vi "DELETE_req_PS.vi"(8 "error in":errorcluster, 10 "URL":string, 11 "Headers":string) -> (0 "error out":errorcluster, 3 "DELETE Request":string)   [LabVIEW 2016]
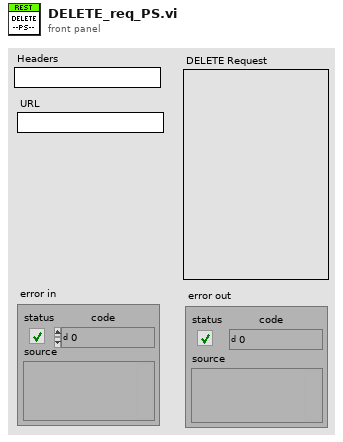
[diagram p1: front panel]
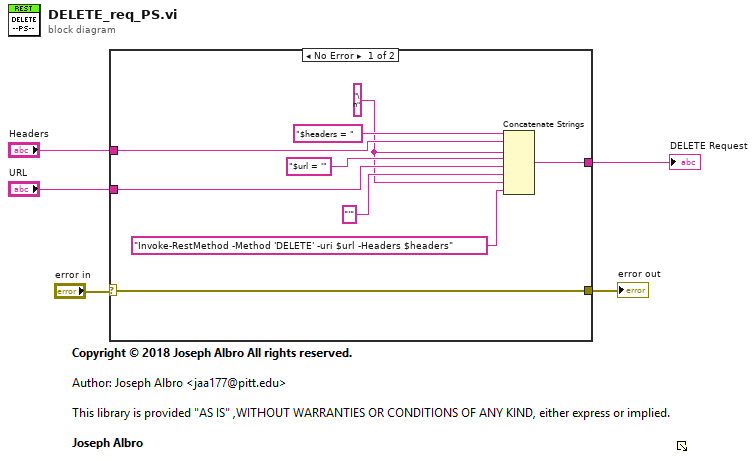
[diagram p0: block diagram]
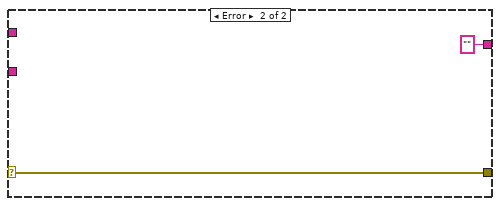
[diagram p2: hidden frame]
diagram:
  n1 = case shown="No Error" "error in" {
    selector: "error in" -> [w6 w15]
    tunnel: "Headers" -> [w14 _]
    tunnel: "URL" -> [w11 _]
    tunnel: [w9 ""] -> w3
    tunnel: [w6 w15] -> w1
    frame No Error {
      w8 = "\n"
      n2 = Concatenate Strings("$headers = ", w14, w8, "$url = '" ("string"), w11, "'" ("string"), w8, "Invoke-RestMethod -Method 'DELETE' -uri $url -Headers $headers" ("string")) -> (w9:string)
    }
    frame Error {
    }
  }
  "DELETE Request" <- w3
  "error out" <- w1
